vi "2d.vi"(6 "data in":T6={"Total counts"=0, "cps"=0.0, "live time"=0.0, "pulser"=0.0, "rare counts"=0.0, "other counts"=0.0, "total run time(sec)"=0.0, "adjusted run time(sec)"=0.0, "17O average"=1.0, "17O current"=1.0}, 8 "error in":errorcluster, 9 "1d state control":T7) -> (4 "data out":T6={"Total counts"=0, "cps"=0.0, "live time"=0.0, "pulser"=0.0, "rare counts"=0.0, "other counts"=0.0, "total run time(sec)"=0.0, "adjusted run time(sec)"=0.0, "17O average"=1.0, "17O current"=1.0})   [LabVIEW 2016]
doc: "uses gated region to gather and parse 1d data"
uses:
  controls/1d/1d state event control.ctl
  spectrum/controls/count control.ctl
  controls/display spectrum.ctl
  pixie2d/controls/1d gate selection.ctl
  Drivers/Pixie4DLL.dll
panel:
  out "run data output 2":T1
  out "number of events":dbl
  out "Run time [s]":dbl
  in  "wait time(milliseconds)":i32=125
  in  "1d gate":T3={"channel number"="", "min"=0.0, "max"=32000.0}
  in  "stop":bool
  in  "number of gated regions":i32=3
  in  "spectrum 2":T4 items=["pulser", "gated region 1", "gated region 2", "gated region 3"]
  in  "spectrum":T4 items=["pulser", "gated region 1", "gated region 2", "gated region 3"]
  out "gate 2":dbl[][](graph)
  out "gate 1":dbl[][](graph)
  out "display array out":T5(array[cluster])
  out "Pixie4DLL calls error":errorcluster
  out "run time":sgl
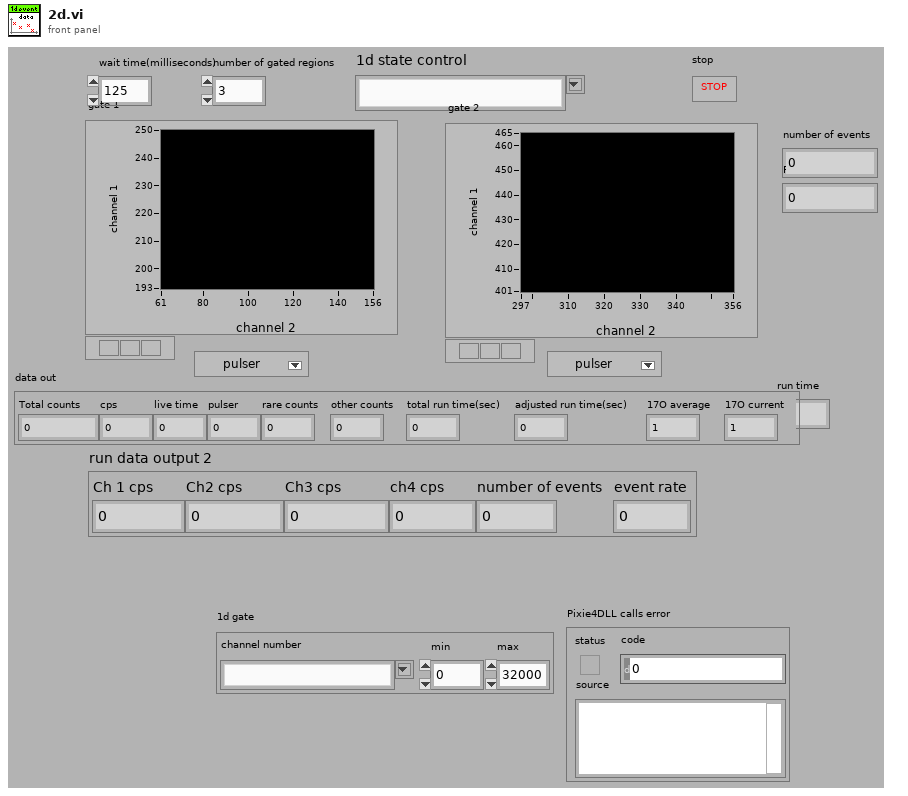
[diagram p1: front panel]
types:
  T1 = cluster{"Ch 1 cps":dbl, "Ch2 cps":dbl, "Ch3 cps":dbl, "ch4 cps":dbl, "number of events":dbl, "event rate":dbl}
  T2 = typedef "1d gate selection.ctl" = string
  T3 = cluster{"channel number":T2, "min":dbl, "max":dbl}
  T4 = typedef "display spectrum.ctl" = u16
  T5 = cluster{"X name":string, "Y name ":string, "counts":dbl, "gate 1":dbl[][], "count rate":dbl, "X Peak":dbl, "Y Peak":dbl, "cathode position":dbl}[]
  T6 = typedef "count control.ctl" = cluster{"Total counts":u32, "cps":dbl, "live time":dbl, "pulser":dbl, "rare counts":dbl, "other counts":dbl, "total run time(sec)":dbl, "adjusted run time(sec)":dbl, "17O average":dbl, "17O current":dbl}
  T7 = typedef "1d state event control.ctl" = string
  T8 = cluster{"X name":string, "Y name ":string, "counts":dbl, "gate 1":dbl[][], "count rate":dbl, "X Peak":dbl, "Y Peak":dbl, "cathode position":dbl}
  T9 = cluster{"input count rate 0":dbl, "input count rate 1":dbl, "input count rate 2":dbl, "input count rate 3":dbl, "number of events":dbl, "event rate":dbl}
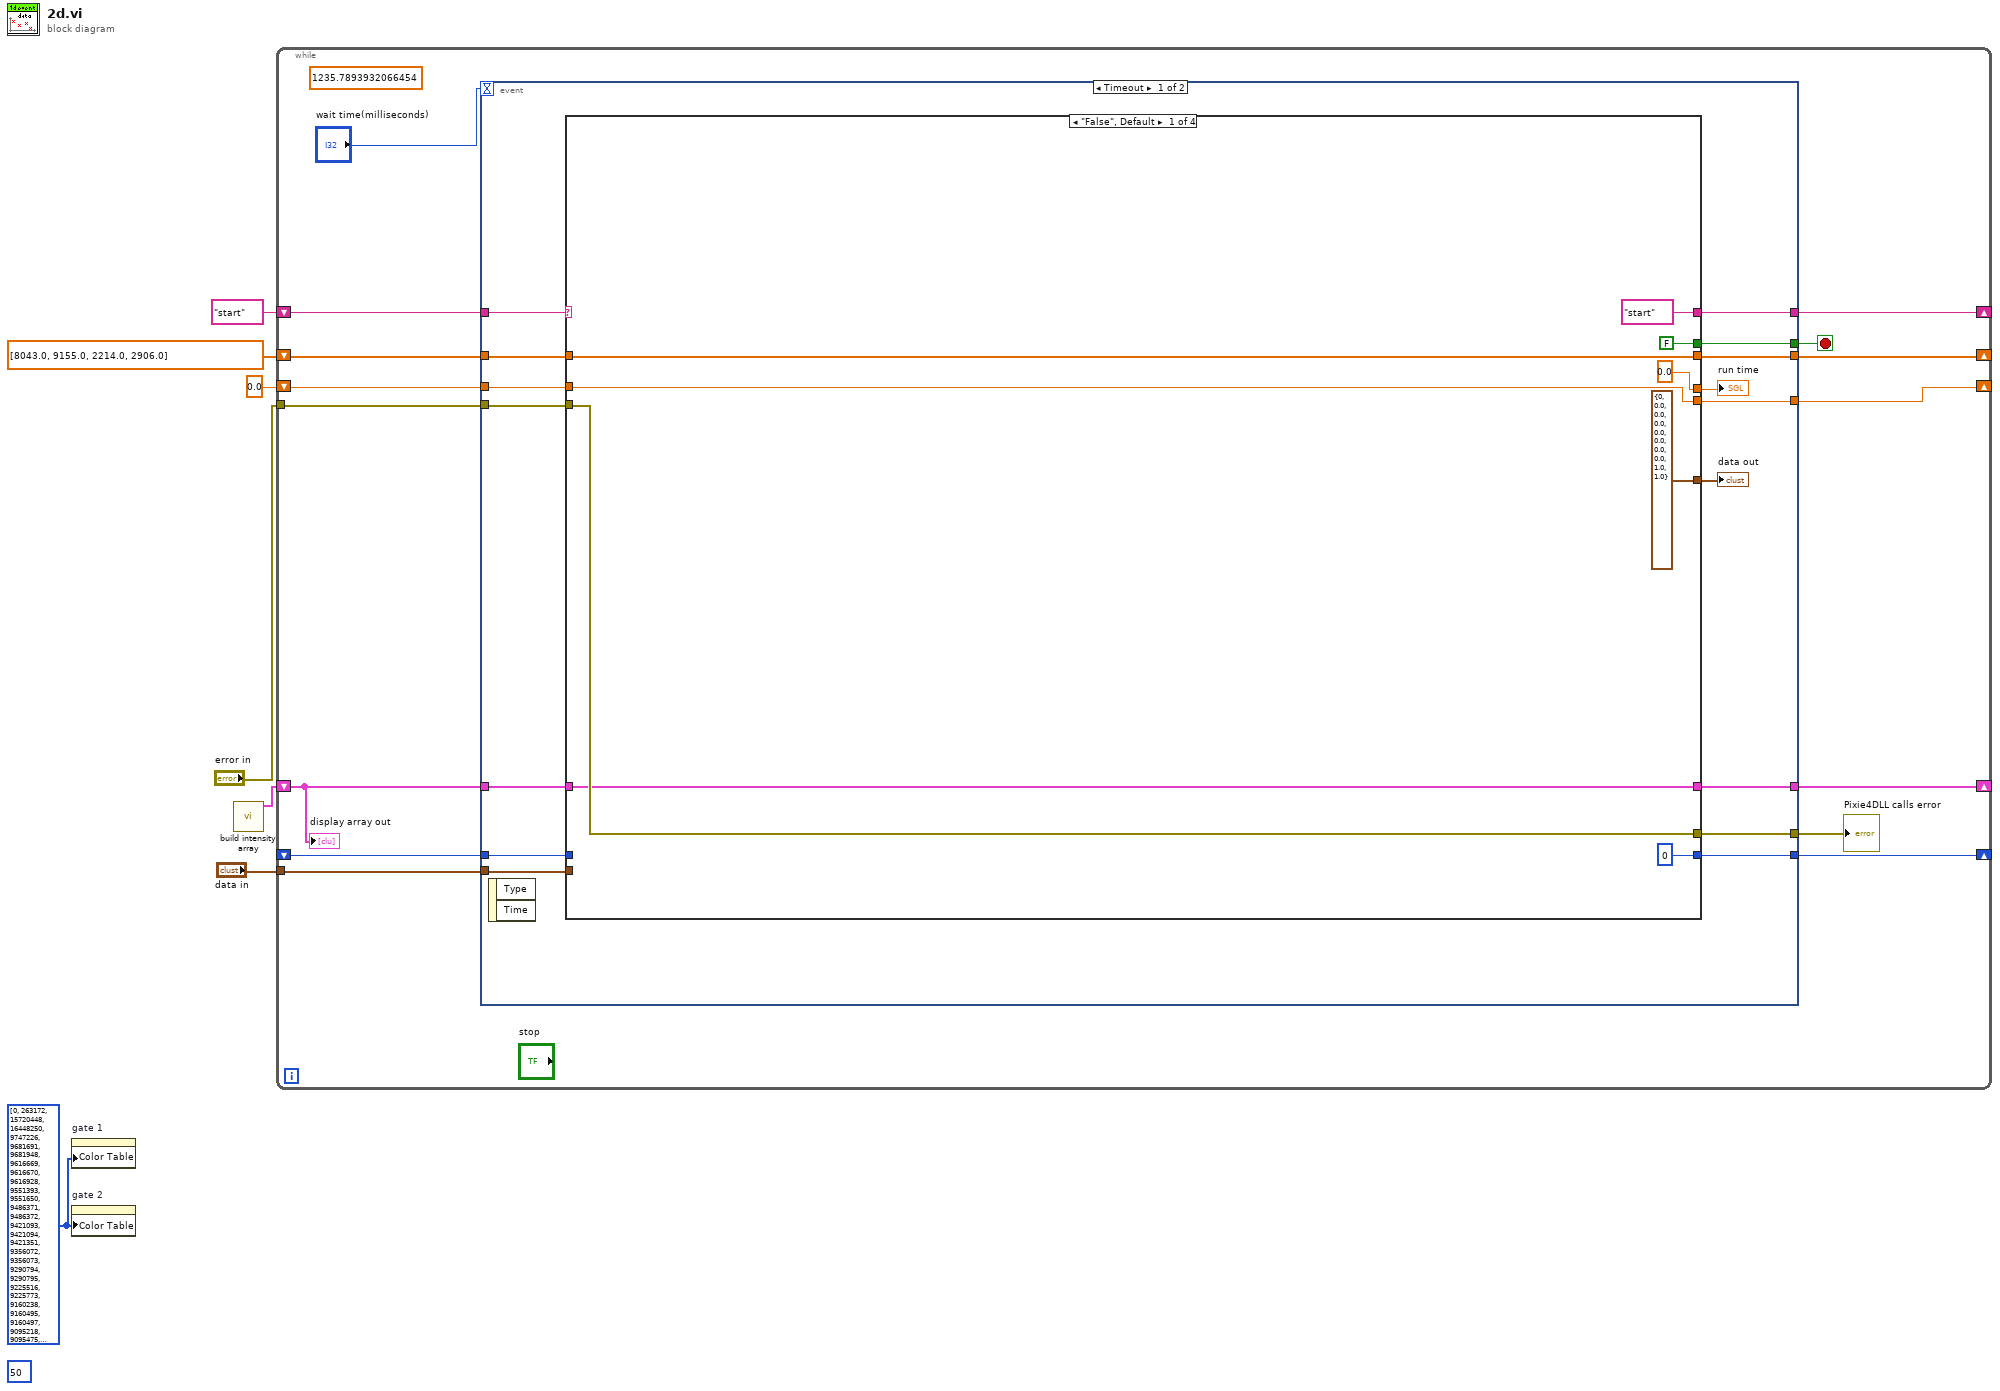
[diagram p0: block diagram]
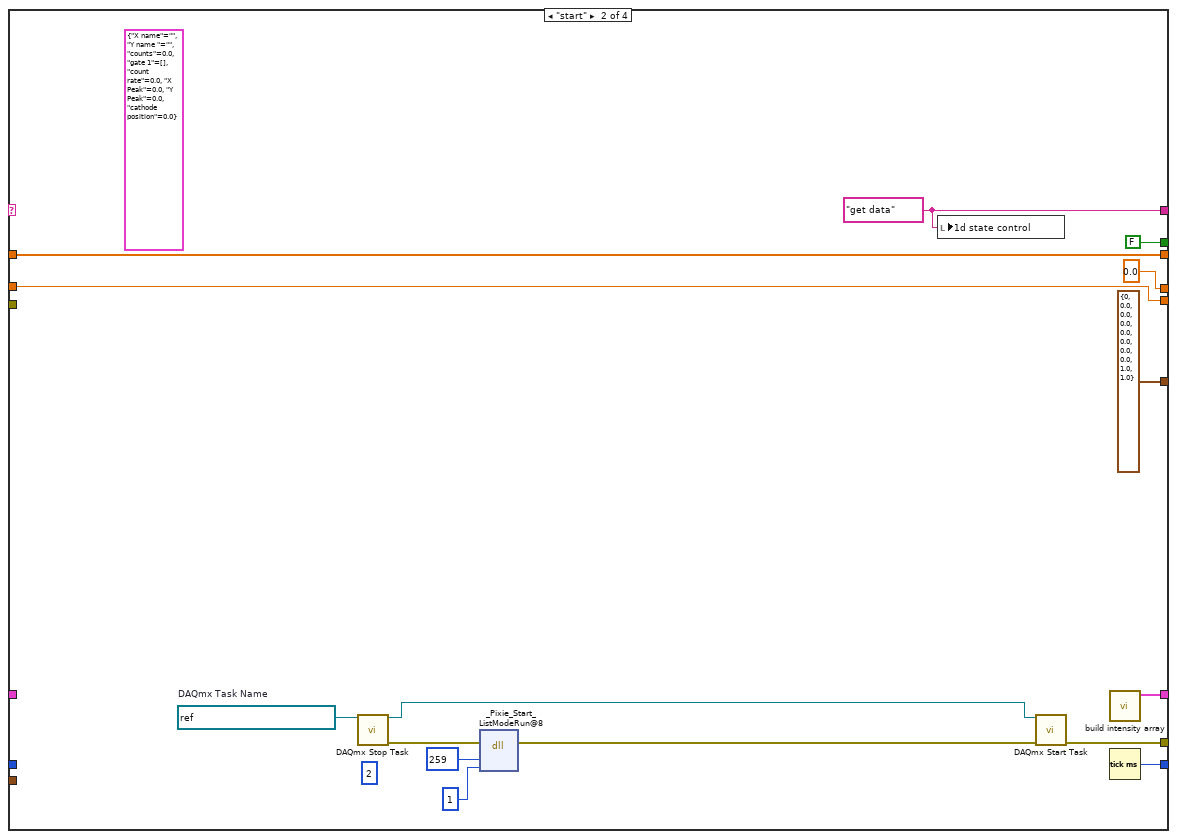
[diagram p2: hidden frame]
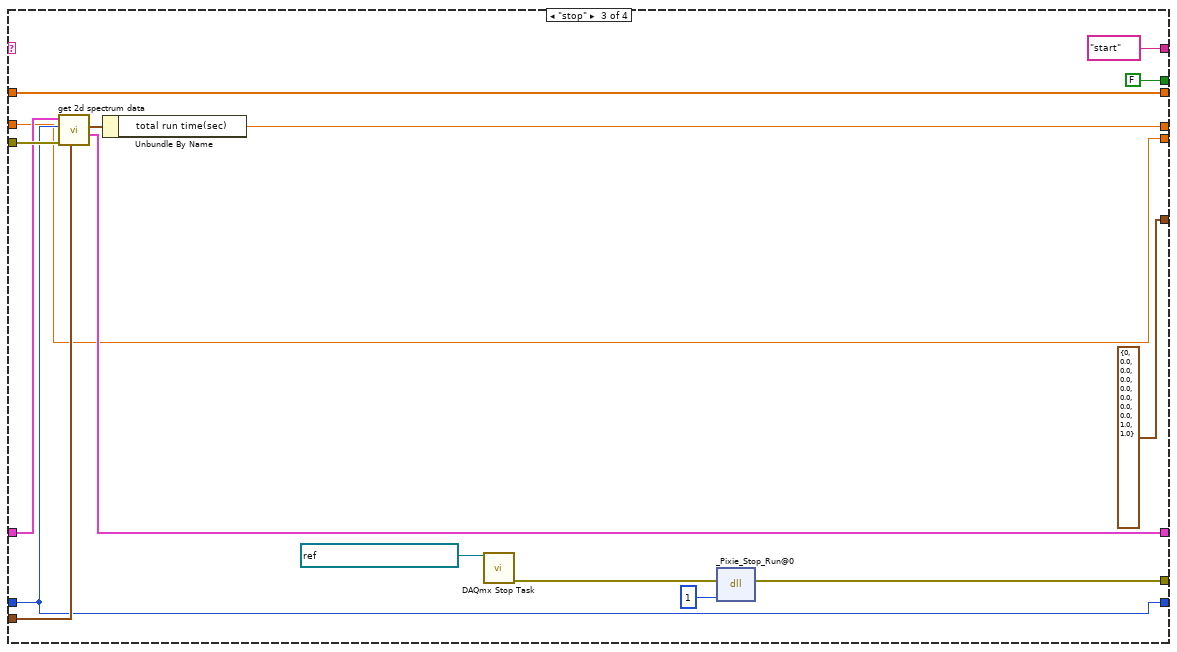
[diagram p3: hidden frame]
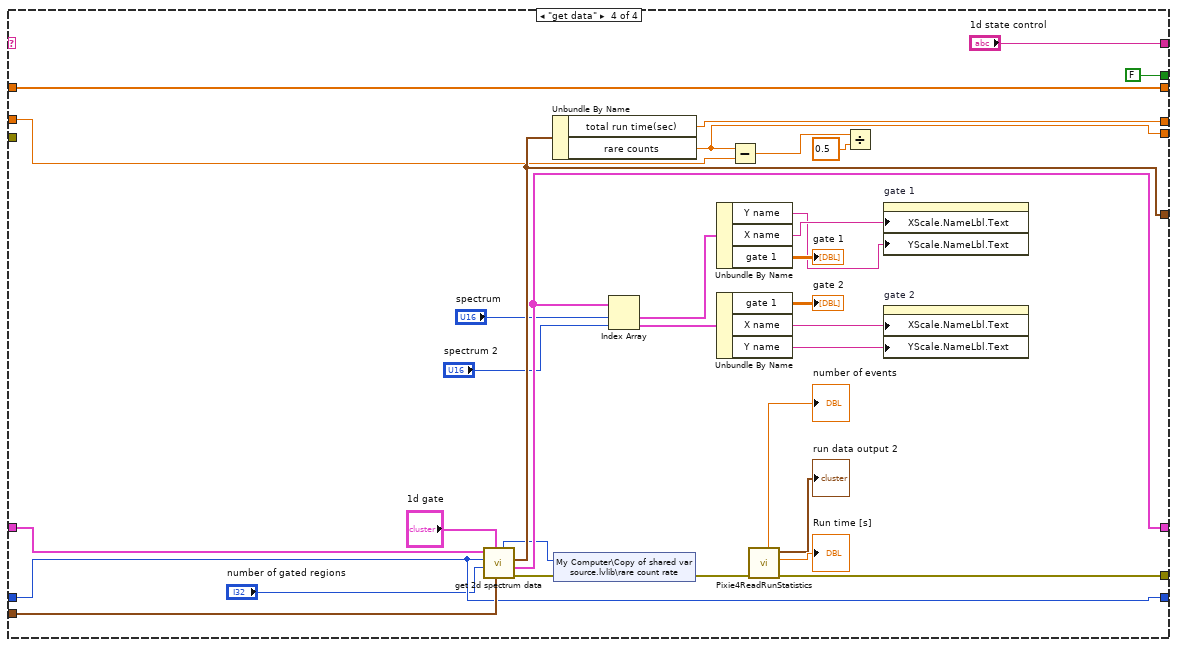
[diagram p4: hidden frame]
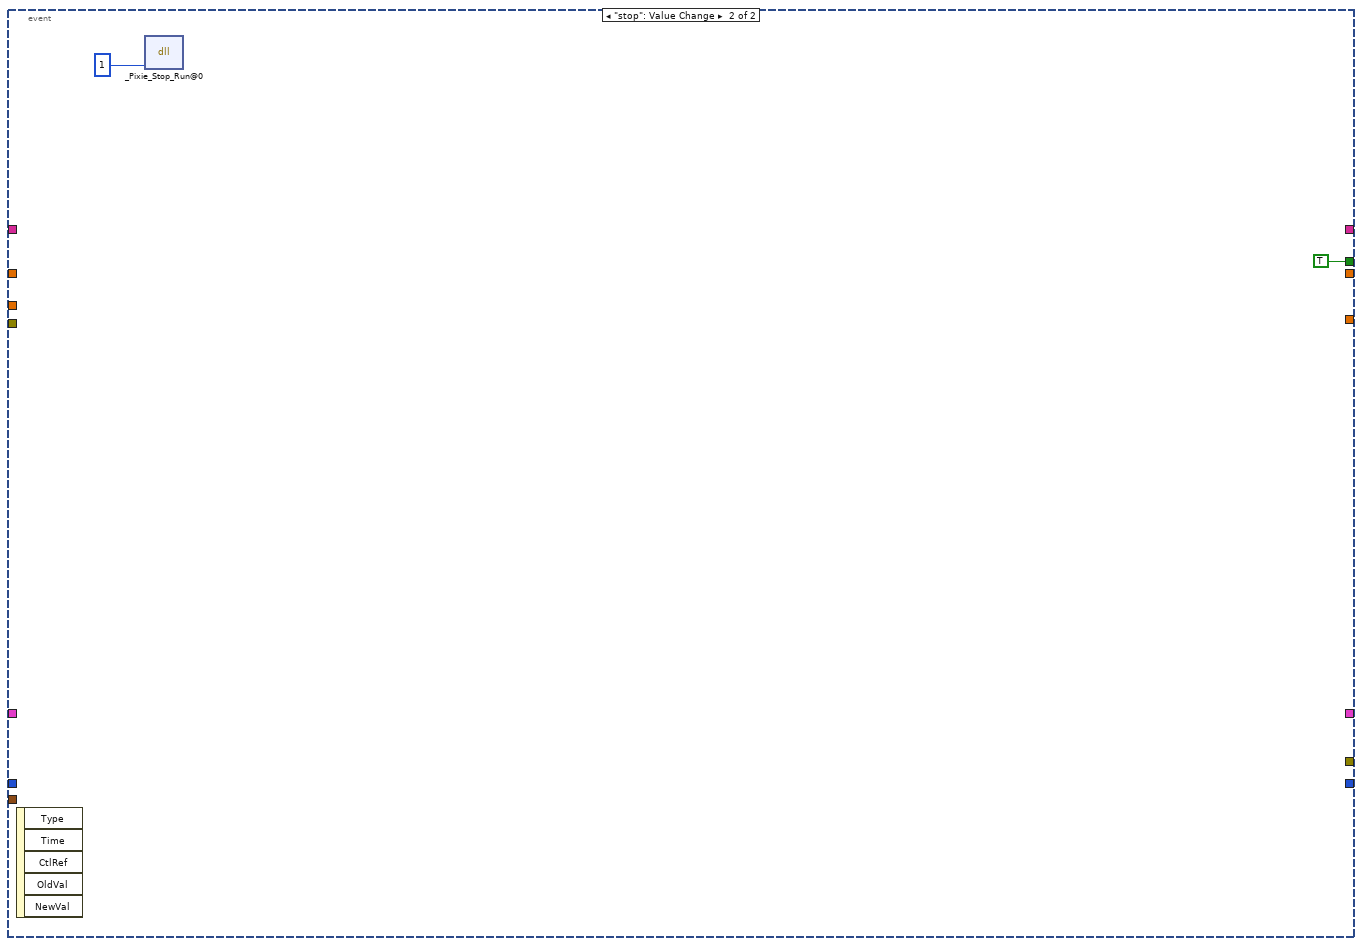
[diagram p5: hidden frame]
diagram:
  w2 = u32[] [0, 263172, 15720448, 16448250, 9747226, 9681691, 9681948, 9616669, 9616670, 9616928, 9551393, 9551650, 9486371, 9486372, 9421093, 9421094, 9421351, 9356072, 9356073, 9290794, 9290795, 9225516, 9225773, 9160238, 9160495, 9160497, 9095218, 9095475, 9029940, 9030197, 8964918, 8964919, 8965176, 8899641, 8899898, 8834619, 8834620, 8769341, 8769342, 8769599, 8704321, 8704322, 8639043, 8639044, 8573765, 8574022, 8574023, 8508744, 8508745, 8443466, 8443723, 8378188, 8378445, 8312910, 8313167, 8312912, 8247122, 8246867, 8181076, 8181077, 8115286, 8115031, 8114776, 8048985, 8048730, 7982939, 7982684, 7916893, 7916894, 7916639, 7850848, 7850594, 7784803, 7784548, 7718757, 7718502, 7718503, 7652712, 7652457, 7586666, 7586411, 7520620, 7520365, 7454574, 7454319, 7454320, 7388529, 7388275, 7322484, 7322229, 7256438, 7256183, 7255928, 7190137, 7190138, 7124347, 7124092, 7058301, 7058046, 7057791, 6992000, 6991745, 6926211, 6925956, 6860165, 6859910, 6859655, 6793864, 6793609, 6727818, 6727563, 6662028, 6661773, 6595982, 6595727, 6595472, 6529681, 6529426, 6463636, 6463381, 6397846, 6397591, 6397336, 6331545, 6331290, 6265499, 6265243, 6199451, 6199451, 6199195, 6133403, 6133147, 6067355, 6067100, 6001308, 6001052, 6000796, 5935260, 5935004, 5869212, 5868956, 5803164, 5802908, 5737116, 5736860, 5736604, 5671068, 5670813, 5605021, 5604765, 5538973, 5538717, 5538461, 5472669, 5472413, 5406877, 5406621, 5340829, 5340573, 5340317, 5274525, 5274270, 5208478, 5208478, 5142686, 5142430, 5142174, 5076382, 5076126, 5010334, 5010078, 4944286, 4944286, 4878494, 4878238, 4877982, 4812191, 4811935, 4746143, 4745887, 4680095, 4680095, 4679839, 4614047, 4613791, 4547999, 4547743, 4481951, 4481695, 4678303, 4874656, 5005472, 5201824, 5398176, 5594528, 5790880, 5987232, 6183584, 6314656, 6511008, 6707360, 6903712, 7100064, 7230880, 7427233, 7623585, 7819937, 8016545, 8212897, 8409249, 8540065, 8736417, 8932769, 9129121, 9325473, 9456545, 9652897, 9849249, 10045601, 10241954, 10438306, 10634658, 10765474, 10961826, 11158434, 11354786, 11551138, 11681954, 11878306, 12074658, 12271010, 12467362, 12663714, 12860323, 12991139, 13187491, 13383843, 13580195, 13776547, 13907363, 14103715, 14300323, 14496675, 14693027, 14889379, 15085731, 15216547, 15412900, 15609252, 15805604, 16002212, 16133028, 16329380, 16525732, 16722084, 16711680, 16448250, 16448250, 16448250]
  (unwired) 50
  n1 = property on="gate 1" class="IntGraph (strict)"("Color Table"=w2) -> ()  [unwired: 2 in, 2 out]
  n2 = property on="gate 2" class="IntGraph (strict)"("Color Table"=w2) -> ()  [unwired: 2 in, 2 out]
  n3 = call "build intensity array.vi"() -> ("display array out"=w3:T5)  [unwired: 10 in, 1 out]
  n4 = while {
    tunnel: "error in" -> [w20]
    tunnel: "data in" -> [w19]
    shift-right: [w18] -> _
    shift-left: _ -> [w22]
    shift-right: [w14] -> _
    shift-left: dbl[] [8043.0, 9155.0, 2214.0, 2906.0] ("Array 2") -> [w21]
    shift-right: [w12] -> _
    shift-left: T7 "start" ("1d state control") -> [w17]
    shift-right: [w11] -> _
    shift-left: w3 -> [w10]
    shift-right: [w9] -> _
    shift-left: 0.0 ("total run time(sec)") -> [w8]
    stop <- w16 stop-if-true
    (unwired) 1235.7893932066454 ("element")
    n5 = event shown="[0] Timeout" {
      selector: _ -> [_ _]
      dyn-events: _ -> [_ _]
      timeout: "wait time(milliseconds)" -> [_ _]
      tunnel: w22 -> [w38 _]
      tunnel: w21 -> [w36 _]
      tunnel: w20 -> [w35 _]
      tunnel: w19 -> [w34 _]
      tunnel: [w33 _] -> w18
      tunnel: [w32 _] -> w14
      tunnel: w17 -> [w31 _]
      tunnel: [w28 TRUE ("stop")] -> w16
      tunnel: [w30 _] -> w15
      tunnel: [w27 _] -> w12
      tunnel: [w26 _] -> w11
      tunnel: w10 -> [w25 _]
      tunnel: [w24 _] -> w9
      tunnel: w8 -> [w23 _]
      event Timeout {
        n6 = event-data() -> ()  [unwired: 1 in, 2 out]
        n7 = case shown="\"False\", Default" w31 {
          tunnel: w38 -> [_ _ w74 w108]
          tunnel: [0.0 0.0 w77 w86] -> w37
          tunnel: w36 -> [w45 w60 w73 w107]
          tunnel: [T6 {"Total counts"=0, "cps"=0.0, "live time"=0.0, "pulser"=0.0, "rare counts"=0.0, "other counts"=0.0, "total run time(sec)"=0.0, "adjusted run time(sec)"=0.0, "17O average"=1.0, "17O current"=1.0} ("data in") T6 {"Total counts"=0, "cps"=0.0, "live time"=0.0, "pulser"=0.0, "rare counts"=0.0, "other counts"=0.0, "total run time(sec)"=0.0, "adjusted run time(sec)"=0.0, "17O average"=1.0, "17O current"=1.0} ("data in") T6 {"Total counts"=0, "cps"=0.0, "live time"=0.0, "pulser"=0.0, "rare counts"=0.0, "other counts"=0.0, "total run time(sec)"=0.0, "adjusted run time(sec)"=0.0, "17O average"=1.0, "17O current"=1.0} ("data in") w110] -> w29
          tunnel: w35 -> [w44 _ w76 _]
          tunnel: w34 -> [_ _ w75 w109]
          tunnel: [u32 0 ("millisecond timer value") w61 w74 w108] -> w33
          tunnel: [w45 w60 w73 w107] -> w32
          tunnel: [w44 w55 w68 w82] -> w30
          tunnel: [FALSE ("stop") FALSE ("stop") FALSE ("stop") FALSE ("stop")] -> w28
          tunnel: [T7 "start" ("1d state control") w57 T7 "start" ("1d state control") "1d state control"] -> w27
          tunnel: [w40 w49 w65 w103] -> w26
          tunnel: w25 -> [w40 _ w64 w104]
          tunnel: [w39 w48 w63 w87] -> w24
          tunnel: w23 -> [w39 w48 w63 w90]
          frame "False", Default {
          }
          frame "start" {
            (unwired) T8 {"X name"="", "Y name "="", "counts"=0.0, "gate 1"=[], "count rate"=0.0, "X Peak"=0.0, "Y Peak"=0.0, "cathode position"=0.0} ("xy position cluster")
            (unwired) 2 ("index")
            w56 = refnum<k21> "MyCountEdgesTask"  # DAQmx Task Name
            w57 = T7 "get data" ("1d state control")
            n8 = call <vilib>:"DAQmx Stop Task.vi"("task/channels in"=w56) -> ("task out"=w52:refnum<k21>, "error out"=w51:errorcluster)  [unwired: 13 in]
            n9 = dll-call lib="D:/Users/wymanm/Desktop/DAQuiri - 2017a/PRIME DAQ 2017a/Drivers/Pixie4DLL.dll" fn="_Pixie_Start_ListModeRun@8"(error in=w51, "Run_Type"=u16 259, "Mode"=1) -> (error out=w50:errorcluster)  [unwired: 2 in, 4 out]
            n10 = local write "1d state control"(w57) -> ()
            n11 = call <vilib>:"DAQmx Start Task.vi"("task/channels in"=w52, "error in"=w50) -> ("error out"=w55:errorcluster)  [unwired: 12 in, 1 out]
            n12 = call "build intensity array.vi"() -> ("display array out"=w49:T5)  [unwired: 10 in, 1 out]
            n13 = Tick Count (ms)() -> (millisecond timer value=w61:u32)
          }
          frame "stop" {
            n14 = call "get 2d spectrum data.vi"("data in"=w75, "error in"=w76, "time in"=w74, "display array in"=w64) -> ("display array out"=w65:T5, "data out"=w67:T6)  [unwired: 2 in, 4 out]
            n15 = Unbundle By Name(w67) -> ("total run time(sec)"=w77:dbl)
            n16 = call <vilib>:"DAQmx Stop Task.vi"("task/channels in"=refnum<k21> "MyCountEdgesTask") -> ("error out"=w69:errorcluster)  [unwired: 13 in, 1 out]
            n17 = dll-call lib="D:/Users/wymanm/Desktop/DAQuiri - 2017a/PRIME DAQ 2017a/Drivers/Pixie4DLL.dll" fn="_Pixie_Stop_Run@0"(error in=w69, "mode"=u16 1 ("ModNum")) -> (error out=w68:errorcluster)  [unwired: 4 in, 1 out]
          }
          frame "get data" {
            n18 = call "get 2d spectrum data.vi"("data in"=w109, "Cluster"="1d gate", "number of gated regions"="number of gated regions", "time in"=w108, "display array in"=w104) -> ("error out"=w98:errorcluster, "display array out"=w103:T5, "data out"=w110:T6, "counts"=w84:u32)  [unwired: 1 in, 2 out]
            n19 = Unbundle By Name(w110) -> ("total run time(sec)"=w86:dbl, "rare counts"=w87:dbl)
            n20 = shared-variable "My Computer\\Copy of shared var source.lvlib\\rare count rate"(w84, error in=w98) -> (error out=w83:errorcluster)
            n21 = Index Array(array=w103, index #1="spectrum", index #2="spectrum 2") -> (element #1=w102:T8, element #2=w101:T8)
            n22 = Unbundle By Name(w102) -> ("Y name"=w93:string, "X name"=w94:string, "gate 1"=→"gate 1":dbl[][])
            n23 = Unbundle By Name(w101) -> ("gate 1"=→"gate 2":dbl[][], "X name"=w92:string, "Y name"=w91:string)
            n24 = Subtract(x=w87, y=w90) -> (x-y=w89:dbl)
            n25 = call "Pixie4ReadRunStatistics.vi"("error in (no error)"=w83) -> ("error out"=w82:errorcluster, "Run time [s]"=→"Run time [s]":dbl, "run data output"=→"run data output 2":T9, "number of events"=→"number of events":dbl)  [unwired: 7 in]
            n26 = Divide(x=w89, y=0.5) -> ()  [unwired: 1 out]
            n27 = property on="gate 1" class="IntGraph (strict)"("XScale.NameLbl.Text"=w94, "YScale.NameLbl.Text"=w93) -> ()  [unwired: 2 in, 2 out]
            n28 = property on="gate 2" class="IntGraph (strict)"("XScale.NameLbl.Text"=w92, "YScale.NameLbl.Text"=w91) -> ()  [unwired: 2 in, 2 out]
          }
        }
        "run time" <- w37
        "data out" <- w29
      }
      event "stop": Value Change {
        n29 = event-data() -> ()  [unwired: 1 in, 5 out]
        n30 = dll-call lib="D:/Users/wymanm/Desktop/DAQuiri - 2017a/PRIME DAQ 2017a/Drivers/Pixie4DLL.dll" fn="_Pixie_Stop_Run@0"("mode"=u16 1 ("ModNum")) -> ()  [unwired: 5 in, 2 out]
      }
    }
    "Pixie4DLL calls error" <- w15
    "display array out" <- w10
  }
